vi "startMasterQueue.vi"(1 "ROS_Master in":refnum<class "ROS_Master.lvclass">) -> (0 "ROS_Master out":refnum<class "ROS_Master.lvclass">)   [LabVIEW 2012, in "ROS_Master.lvclass"]
uses:
  ROS_Master.lvclass
  ROS_Master.lvclass/ROS_Master.ctl
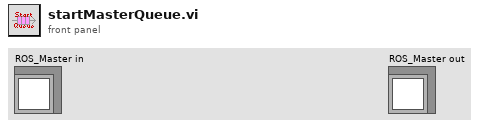
[diagram p1: front panel]
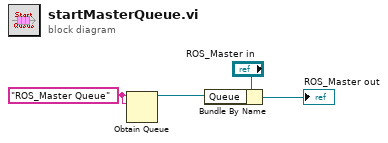
[diagram p0: block diagram]
diagram:
  w2 = "ROS_Master Queue" ("name (unnamed)")
  n1 = Obtain Queue(name (unnamed)=w2, element data type=w2) -> (queue out=w1:refnum<queue>)  [unwired: 3 in, 2 out]
  n2 = Bundle By Name(cluster="ROS_Master in", "Queue"=w1) -> (→"ROS_Master out":refnum<class "ROS_Master.lvclass">)
